vi "Stat_plane.vi"(11 "HOLO_array":sgl[][](array[numeric])) -> (3 "String":string)   [LabVIEW 2023]
uses:
  <vilib>/Analysis/NI_AALBase.lvlib
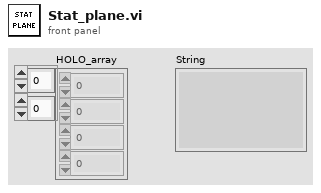
[diagram p1: front panel]
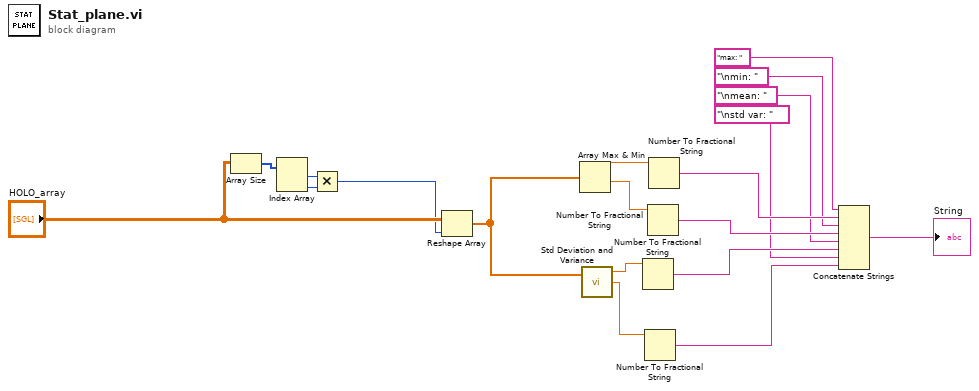
[diagram p0: block diagram]
diagram:
  n1 = Array Size(array="HOLO_array") -> (size(s)=w4:i32[])
  n2 = Index Array(array=w4) -> (element #1=w3:i32, element #2=w2:i32)  [unwired: 2 in]
  n3 = Multiply(x=w3, y=w2) -> (x*y=w1:i32)
  n4 = Reshape Array("HOLO_array", w1) -> (w19:sgl[])
  n5 = Array Max & Min(array=w19) -> (max value=w18:sgl, min value=w17:sgl)  [unwired: 2 out]
  n6 = call <vilib>:"Std Deviation and Variance.vi"("X"=w19) -> ("mean"=w16:dbl, "standard deviation"=w15:dbl)  [unwired: 1 in, 1 out]
  n7 = Number To Fractional String(number=w16) -> (F-format string=w9:string)  [unwired: 3 in]
  n8 = Number To Fractional String(number=w15) -> (F-format string=w7:string)  [unwired: 3 in]
  n9 = Number To Fractional String(number=w17) -> (F-format string=w11:string)  [unwired: 3 in]
  n10 = Number To Fractional String(number=w18) -> (F-format string=w13:string)  [unwired: 3 in]
  n11 = Concatenate Strings("max: ", w13, "\nmin: ", w11, "\nmean: ", w9, "\nstd var: ", w7) -> (→"String":string)
